vi "Initialize Waveforms V1.vi"() -> ()   [LabVIEW 2014]
uses:
  Type Defs/Image Acquisition Parameters.ctl
  <vilib>/Analysis/NI_AALPro.lvlib
  <vilib>/Analysis/2dsp.llb/1D Convolution (DBL).vi
panel:
  out "XY Graph":cluster{i32[], dbl[]}(graph)
  in  "um to Volts Conversion":dbl
  in  "Max Speed (v/s)":dbl
  in  "Width":dbl
  in  "Image Acquisition Parameters":T1={"Scan Type"=enum."Sample Scanning", "Scan Mode"=enum."XY", "Fast Axis Frequency (Hz)"=100.0, "Image Format"=128, "Field of View (um)"=0.0, "Line Accumulations"=0.0} {"Image Format" items=["64 x 64"=64, "128 x 128"=128, "256 x 256"=256, "512 x 512"=512, "1024 x 1024"=1024, "2048 x 2048"=2048]}
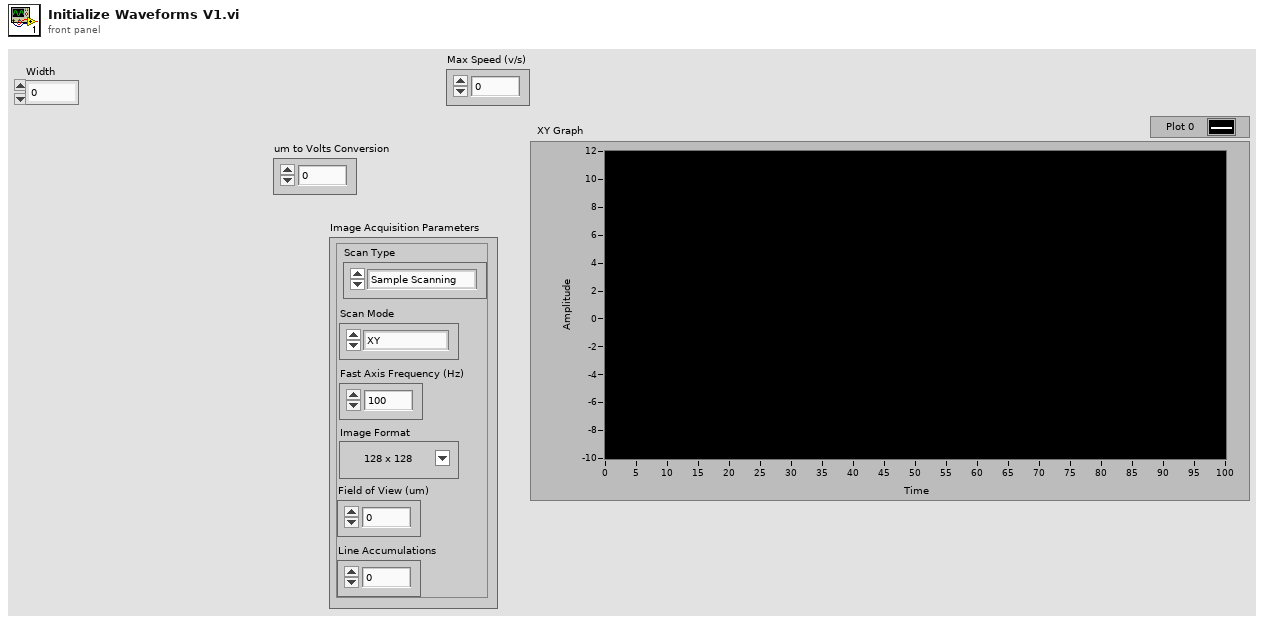
[diagram p1: front panel]
types:
  T1 = typedef "Image Acquisition Parameters.ctl" = cluster{"Scan Type":enum16{"Sample Scanning", "Beam Scanning"}, "Scan Mode":enum16{"XY", "XZ", "YZ", "XYZ"}, "Fast Axis Frequency (Hz)":dbl, "Image Format":u16, "Field of View (um)":dbl, "Line Accumulations":dbl}
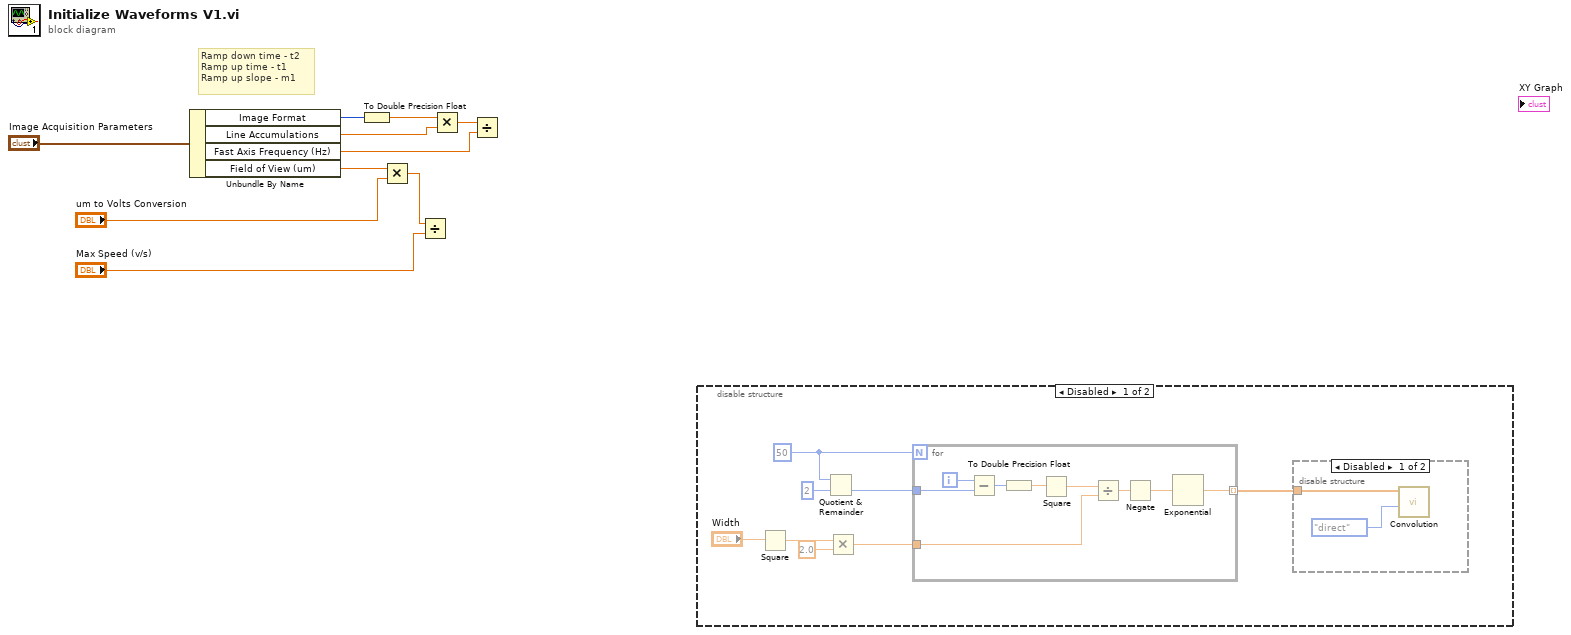
[diagram p0: block diagram]
diagram:
  # "Ramp down time - t2\nRamp up time - t1\nRamp up slope - m1"
  n1 = Unbundle By Name("Image Acquisition Parameters") -> ("Image Format"=w9:u16, "Line Accumulations"=w8:dbl, "Fast Axis Frequency (Hz)"=w7:dbl, "Field of View (um)"=w6:dbl)
  n2 = To Double Precision Float(number=w9) -> (double precision float=w3:dbl)
  n3 = Multiply(x=w6, y="um to Volts Conversion") -> (x*y=w1:dbl)
  n4 = Divide(x=w1, y="Max Speed (v/s)") -> ()  [unwired: 1 out]
  n5 = Multiply(x=w3, y=w8) -> (x*y=w2:dbl)
  n6 = Divide(x=w2, y=w7) -> ()  [unwired: 1 out]
  n7 = disable-structure shown="Disabled" {
    frame Disabled {
      w18 = 50
      n8 = Square(x="Width") -> (x^2=w12:dbl)
      n9 = Quotient & Remainder(x=w18, y=2) -> (floor(x/y)=w16:i32)  [unwired: 1 out]
      n10 = Multiply(x=w12, y=2.0) -> (x*y=w13:dbl)
      n11 = for {
        N: w18 -> [_]
        tunnel: w16 -> [w28]
        tunnel: w13 -> [w24]
        tunnel: [w21] -> w11 mode=indexing
        i -> [w29]
        n12 = Subtract(x=w29, y=w28) -> (x-y=w27:i32)
        n13 = To Double Precision Float(number=w27) -> (double precision float=w26:dbl)
        n14 = Square(x=w26) -> (x^2=w25:dbl)
        n15 = Divide(x=w25, y=w24) -> (x/y=w23:dbl)
        n16 = Negate(x=w23) -> (-x=w22:dbl)
        n17 = Exponential(1:w22) -> (0:w21:dbl)
      }
      n18 = disable-structure shown="Disabled" {
        disable-tunnel: w11 -> [w20 _]
        frame Disabled {
          n19 = call-poly <vilib>:"Convolution.vi"("algorithm"=enum32{"direct", "frequency domain"}."direct", "X"=w20) -> ()  [unwired: 8 in, 2 out]
        }
        frame Enabled {
        }
      }
    }
    frame Enabled {
    }
  }
